vi "JSONRPC_Example.vi"() -> ()   [LabVIEW 2021]
uses:
  <vilib>/NI/JSON Support for LabVIEW/JSON Value/JSON Types.ctl
  <vilib>/NI/JSON Support for LabVIEW/JSON Value/New JSON Value/New JSON (String).vi
  <vilib>/NI/JSON Support for LabVIEW/JSON Value/New JSON Value/New JSON (Numeric).vi
  <vilib>/NI/JSON Support for LabVIEW/JSON Value/New JSON Value/New JSON ({Value[]}).vi
  <vilib>/NI/JSON Support for LabVIEW/JSON Value/JSON Value.lvclass
panel:
  in  "Tab Control":enum32{"Creating", "Parsing"}(tab)
  in  "params":dbl
  in  "method":string
  in  "jsonrpc":string
  out "JSON":string
  in  "Keys":string[](array[string])
  in  "JSON string":string=" {\n \"jsonrpc\": \"2.0\",\n  \"result\": {\n    \"description\": \"9f5449534443495430002f7d3c0139f7\",\n    \"status\": \"Ok\"\n  },\n  \"id\": 0\n}"
  out "keys":string[](array[string])
  out "Values":string[](array[string])
  out "datatype":T1
  # "Values"
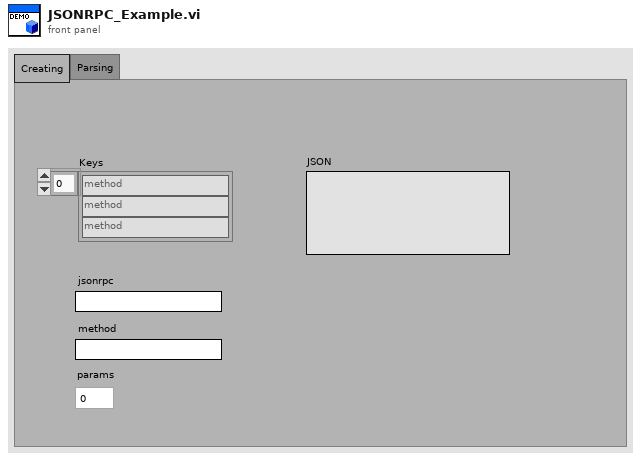
[diagram p1: front panel]
types:
  T1 = typedef "JSON Value.lvclass/JSON Types.ctl" = enum16{"String", "Numeric", "Boolean", "NULL", "Object", "Array"}
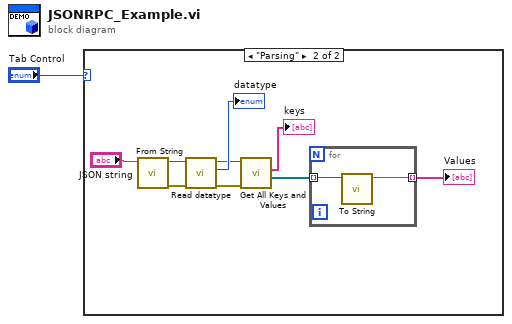
[diagram p0: block diagram]
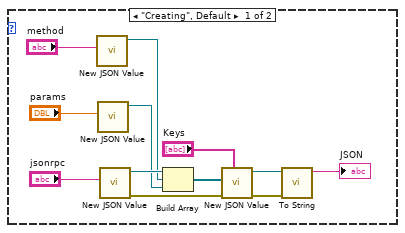
[diagram p2: hidden frame]
diagram:
  n1 = case shown="\"Parsing\"" "Tab Control" {
    frame "Creating", Default {
      n2 = call-poly <vilib>:"New JSON Value.vi"("value"="method") -> ("JSON Value out"=w6:refnum<class "JSON Value.lvclass">)  [unwired: 9 in, 1 out]
      n3 = call-poly <vilib>:"New JSON Value.vi"("value"="params") -> ("JSON Value out"=w7:refnum<class "JSON Value.lvclass">)  [unwired: 9 in, 1 out]
      n4 = call-poly <vilib>:"New JSON Value.vi"("value"="jsonrpc") -> ("error out"=w10:errorcluster, "JSON Value out"=w12:refnum<class "JSON Value.lvclass">)  [unwired: 9 in]
      n5 = Build Array(w12, w6, w7) -> (w11:refnum<class "JSON Value.lvclass">[])
      n6 = call-poly <vilib>:"New JSON Value.vi"("keys"="Keys", "error in (no error)"=w10, "values"=w11) -> ("error out"=w8:errorcluster, "JSON Value out"=w9:refnum<class "JSON Value.lvclass">)  [unwired: 7 in]
      n7 = call <vilib>:"To String.vi"("error in (no error)"=w8, "JSON Value in"=w9) -> ("String"=→"JSON":string)  [unwired: 8 in, 1 out]
    }
    frame "Parsing" {
      n8 = call <vilib>:"From String.vi"("JSON String"="JSON string") -> ("error out"=w16:errorcluster, "JSON Value out"=w20:refnum<class "JSON Value.lvclass">)  [unwired: 9 in]
      n9 = call <vilib>:"Read datatype.vi"("error in (no error)"=w16, "JSON Value in"=w20) -> ("error out"=w15:errorcluster, "datatype"=→"datatype":T1, "JSON Value out"=w14:refnum<class "JSON Value.lvclass">)  [unwired: 7 in]
      n10 = call <vilib>:"Get All Keys and Values.vi"("error in"=w15, "JSON Value in"=w14) -> ("values"=w18:refnum<class "JSON Value.lvclass">[], "keys"=→"keys":string[])  [unwired: 7 in, 1 out]
      n11 = for {
        tunnel: w18 -> [w23] mode=indexing
        tunnel: [w24] -> w21 mode=indexing
        n12 = call <vilib>:"To String.vi"("JSON Value in"=w23) -> ("String"=w24:string)  [unwired: 9 in, 1 out]
      }
      "Values" <- w21
    }
  }
